vi "SUNION.vi"(0 "refnum in":refnum<vi>, 1 "Keys":string[](array[string]), 11 "error in":errorcluster) -> (4 "refnum out":refnum<vi>, 6 "Data":T1, 15 "error out":errorcluster)   [LabVIEW 2023]
uses:
  SubVIs/Controls/redis-data.ctl
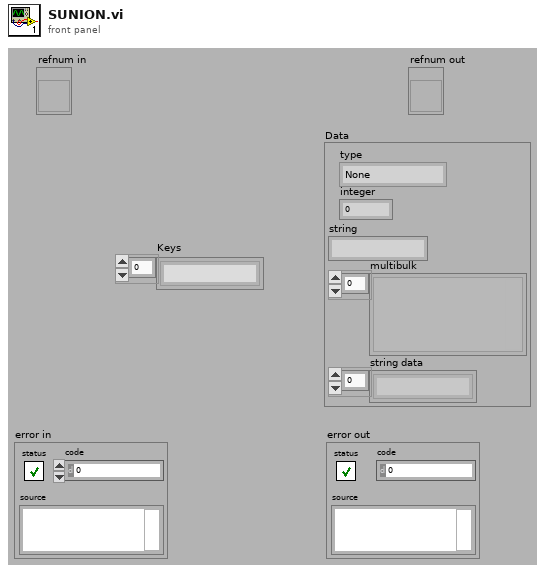
[diagram p1: front panel]
types:
  T1 = typedef "redis-data.ctl" = cluster{"type":enum16{"None", "Error", "Status", "Nil", "Integer", "String", "Multibulk"}, "integer":i64, "string":string, "multibulk":variant[], "string data":string[]}
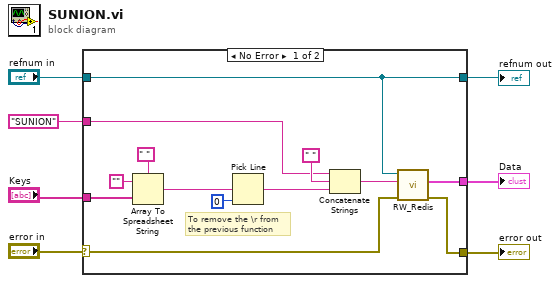
[diagram p0: block diagram]
diagram:
  n1 = case shown="No Error" "error in" {
    selector: "error in" -> [w11 w22]
    tunnel: "Keys" -> [w20 _]
    tunnel: "SUNION" -> [w13 _]
    tunnel: "refnum in" -> [w8 w21]
    tunnel: [w10 w22] -> w3
    tunnel: [w9 _] -> w2
    tunnel: [w8 w21] -> w1
    frame No Error {
      # "To remove the \\r from\nthe previous function"
      n2 = Array To Spreadsheet String(delimiter (Tab)=" ", array=w20, 3:"" ("format string")) -> (spreadsheet string=w15:string)
      n3 = Pick Line(multi-line string=w15, line index=0) -> (output string=w16:string)  [unwired: 1 in]
      n4 = Concatenate Strings(w13, " ", w16) -> (w12:string)
      n5 = call "RW_Redis.vi"("error in"=w11, "command"=w12, "TCP session in"=w8) -> ("error out"=w10:errorcluster, "Data"=w9:T1)  [unwired: 6 in, 1 out]
    }
    frame Error {
    }
  }
  "error out" <- w3
  "Data" <- w2
  "refnum out" <- w1
